vi "TCP-Com.vi"(8 "Exit Control Label":string="Exit Button", 9 "pwd":string, 10 "LabView Port":u16=4000, 11 "VI Refnum":refnum<vi>) -> (0 "error out":errorcluster)   [LabVIEW 2019]
doc: "This template is for the Queued Message Handler design pattern.\n\nThe Event Handling Loop generates messages based on user interface actions.\n\nThe Message Handling Loop processes messages generated by the Event Handling Loop, or by other messages. The messages are string values, so new messages can be added easily to the Message Cases case structure in the Message Handling Loop. Each message cluster can also provide an optional value for Message Data, which is a variant that can be converted to whatever message-specific data is required."
uses:
  support/TPC-Enum.ctl
  support/Message Queue/Enqueue Message (Single).vi
  <vilib>/Utility/error.llb/Error Cluster From Error Code.vi
  <vilib>/ErrorRing/Error Ring.xnode
  support/Message Queue/Message Queue.lvlib
  support/User Event - Stop/User Event - Stop.lvlib
  <vilib>/Utility/Data Type/NI_Data Type.lvlib
panel:
  out "connection ID":refnum<k5>
  out "Client Connected":bool
  in  "Request":string
  in  "Try request":bool
  in  "Exit":bool
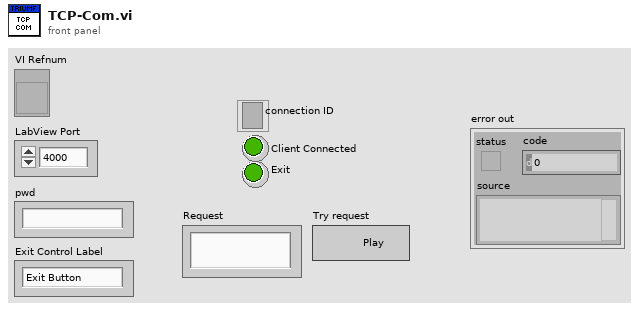
[diagram p1: front panel]
types:
  T1 = typedef "TPC-Enum.ctl" = enum16{"Wait For Client", "Check Client", "Listen"}
  T2 = typedef "Message Queue.lvlib/All Message Queues.ctl" = cluster{"TCP":refnum<queue>}
  T3 = typedef "NI_Data Type.lvlib/Data Type.ctl" = enum8{"Invalid Type", "Void", "I8", "I16", "I32", "I64", "U8", "U16", "U32", "U64", "Single Float", "Double Float", "Extended Float", "Single Complex", "Double Complex", "Extended Complex", "Enum U8", "Enum U16", "Enum U32", "Enum U64", "Single Float With Unit", "Double Float With Unit", "Extended Float With Unit", "Single Complex with Unit", "Double Complex with Unit", "Extended Complex with Unit", "Boolean", "String", "Path", "Picture", "Tag", "Array", "Cluster", "Variant", "LV Variant", "Waveform", "Timestamp", "Digital Waveform", "Digital Data", "ExpressData", "Refnum", "External Data", "VI", "Poly VI", "LabVIEW Class Instance", "Fixed Point", "Set Collection", "Map Collection"}
  T4 = enum16{"Standard", "Buffered", "CRLF", "Immediate"}
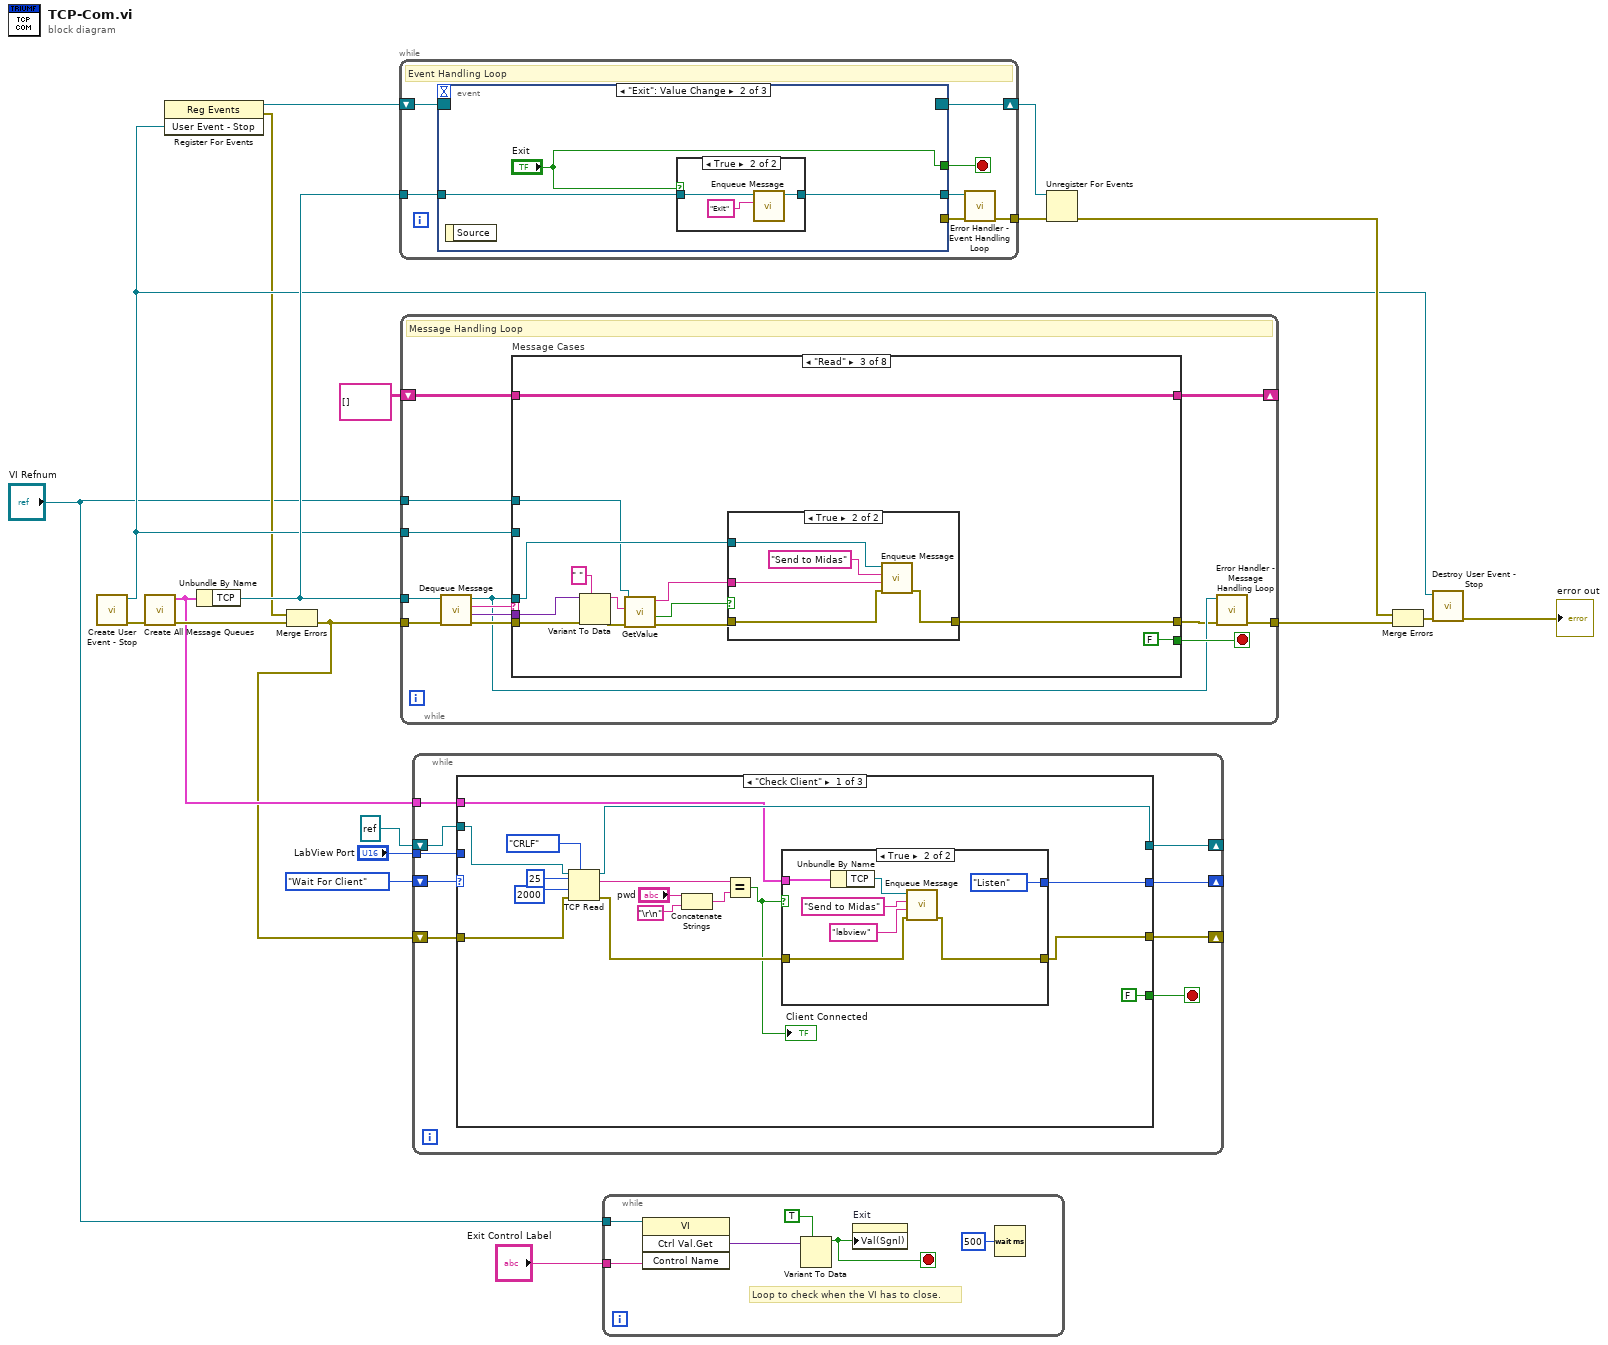
[diagram p0: block diagram]
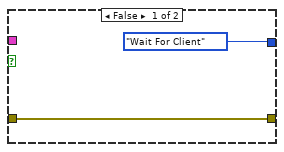
[diagram p2: hidden frame]
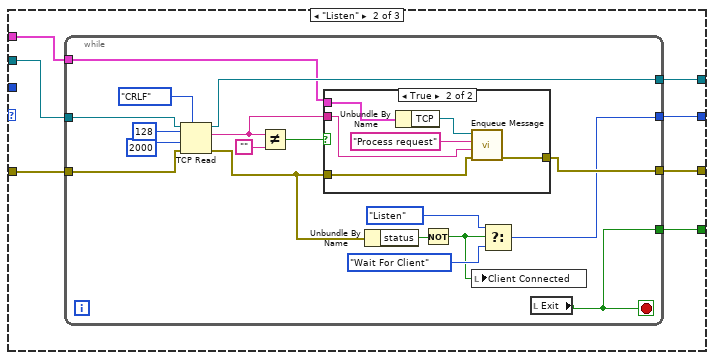
[diagram p3: hidden frame]
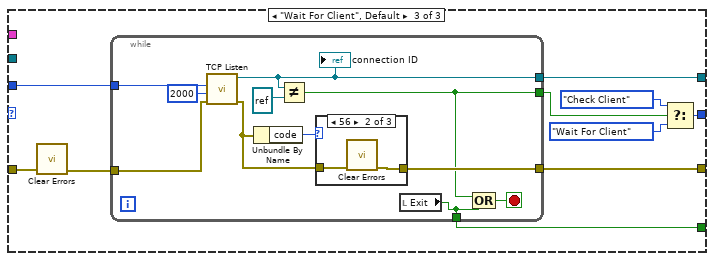
[diagram p5: hidden frame]
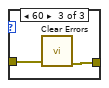
[diagram p7: hidden frame]
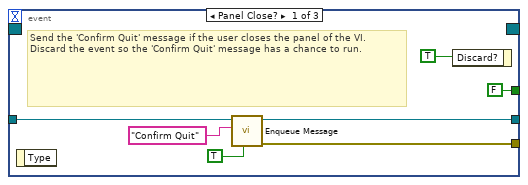
[diagram p8: hidden frame]
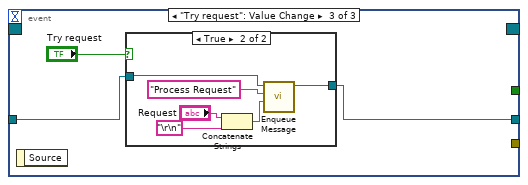
[diagram p10: hidden frame]
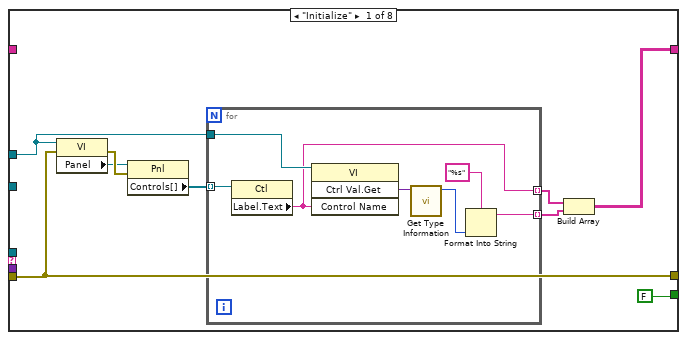
[diagram p12: hidden frame]
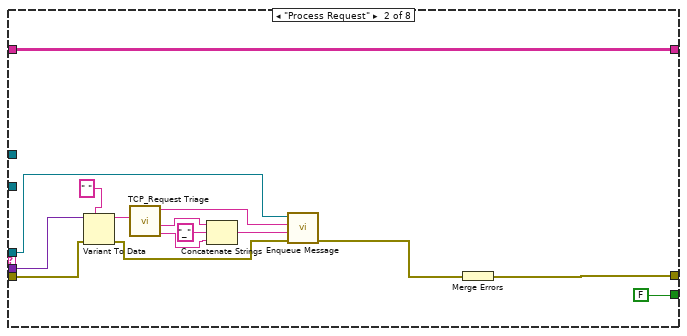
[diagram p13: hidden frame]
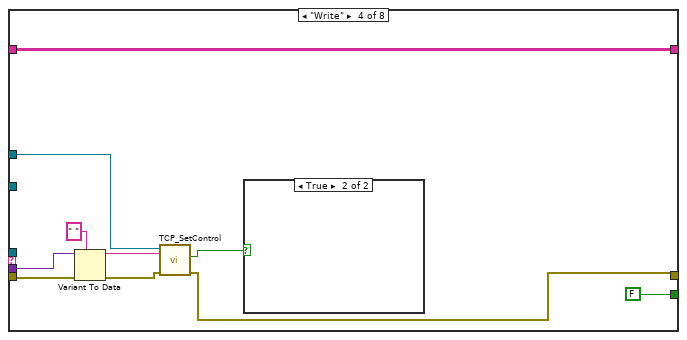
[diagram p15: hidden frame]
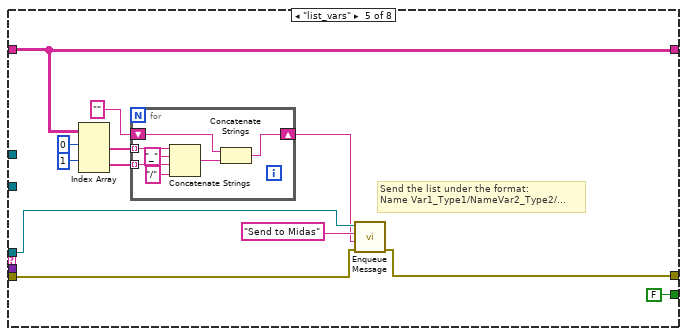
[diagram p17: hidden frame]
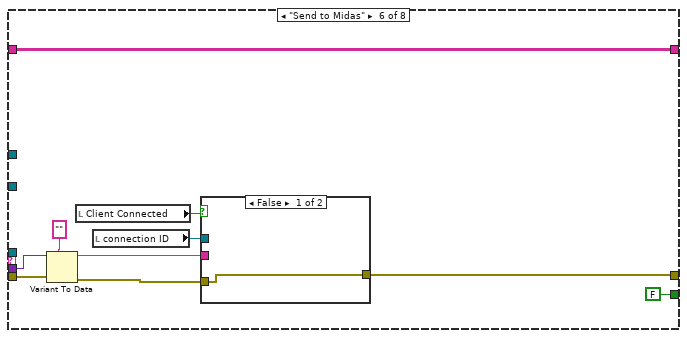
[diagram p18: hidden frame]
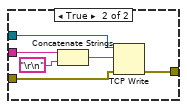
[diagram p19: hidden frame]
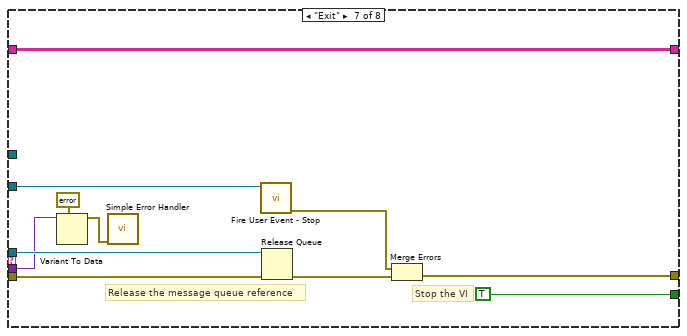
[diagram p20: hidden frame]
diagram:
  n1 = call "Create User Event - Stop.vi"() -> ("error out"=w17:errorcluster, "User Event - Stop"=w11:refnum<user-event>)  [unwired: 10 in]
  n2 = call "Create All Message Queues.vi"("error in (no error)"=w17) -> ("error out"=w20:errorcluster, "Message Queues out"=w6:T2)  [unwired: 9 in]
  n3 = register-events(w11) -> (reference out=w12:refnum<event-registration>, error out=w10:errorcluster)  [unwired: 2 in]
  n4 = Unbundle By Name(w6) -> ("TCP"=w18:refnum<queue>)
  n5 = Merge Errors(w10, w20) -> (w2:errorcluster)
  n6 = while {
    tunnel: w18 -> [w27]
    shift-right: [w25] -> w14
    shift-left: w12 -> [w26]
    tunnel: [w21] -> w13
    stop <- w23 stop-if-true
    # "Event Handling Loop"
    n7 = event shown="[1] \"Exit\": Value Change" {
      selector: w26 -> [_ _ _]
      dyn-events: [_ _ _] -> w25
      timeout: _ -> [_ _ _]
      tunnel: [FALSE ("Discard?") "Exit" _] -> w23
      tunnel: w27 -> [w33 w37 w43]
      tunnel: [w32 _ _] -> w24
      tunnel: [w31 w36 w42] -> w22
      event Panel Close? {
        # "Send the 'Confirm Quit' message if the user closes the panel of the VI. Discard the event so the 'Confirm Quit' message has a chance to run."
        n8 = event-data() -> ()  [unwired: 1 in, 1 out]
        n9 = call-poly "Enqueue Message.vi"("Priority Message? (F)"=TRUE, "Message"="Confirm Quit", "Message Queue"=w33) -> ("error out"=w32:errorcluster, "dup Message Queue"=w31:refnum<queue>)  [unwired: 7 in]
        n10 = event-data("Discard?"=TRUE) -> ()  [unwired: 1 in, 1 out]
      }
      event "Exit": Value Change {
        n11 = event-data() -> ()  [unwired: 1 in, 1 out]
        n12 = case shown="True" "Exit" {
          tunnel: w37 -> [w38 w41]
          tunnel: [w38 w39] -> w36
          frame False {
          }
          frame True {
            n13 = call-poly "Enqueue Message.vi"("Message"="Exit", "Message Queue"=w41) -> ("dup Message Queue"=w39:refnum<queue>)  [unwired: 8 in, 1 out]
          }
        }
      }
      event "Try request": Value Change {
        n14 = event-data() -> ()  [unwired: 1 in, 1 out]
        n15 = case shown="True" "Try request" {
          tunnel: w43 -> [w45 w50]
          tunnel: [w45 w49] -> w42
          frame False {
          }
          frame True {
            n16 = Concatenate Strings("Request", "\r\n") -> (w47:string)
            n17 = call-poly "Enqueue Message.vi"("Message Data"=w47, "Message"="Process Request", "Message Queue"=w50) -> ("dup Message Queue"=w49:refnum<queue>)  [unwired: 7 in, 1 out]
          }
        }
      }
    }
    n18 = call "Error Handler - Event Handling Loop.vi"("error in (no error)"=w24, "Message Queue"=w22) -> ("dup error in"=w21:errorcluster)  [unwired: 8 in, 1 out]
  }
  n19 = while {
    tunnel: w18 -> [w58]
    tunnel: w11 -> [w63]
    tunnel: w2 -> [w62]
    tunnel: [w56] -> w19
    tunnel: "VI Refnum" -> [w54]
    shift-right: [w53] -> _
    shift-left: string[][] [] -> [w52]
    stop <- w64 stop-if-true
    # "Message Handling Loop"
    n20 = call "Dequeue Message.vi"("error in (no error)"=w62, "Message Queue"=w58) -> ("error out"=w61:errorcluster, "Message Data"=w59:variant, "Message"=w60:string, "dup Message Queue"=w57:refnum<queue>)  [unwired: 6 in]
    n21 = case "Message Cases" shown="\"Read\"" w60 {
      selector: w60 -> [_ _ _ _ _ _ _ w174]
      tunnel: w57 -> [_ w88 w105 _ w135 _ w171 _]
      tunnel: w61 -> [w69 w93 w107 w123 w134 w151 w165 _]
      tunnel: [w69 w95 w104 w115 w133 w144 w168 w175] -> w55
      tunnel: [FALSE FALSE FALSE FALSE FALSE FALSE TRUE FALSE] -> w64
      tunnel: w59 -> [_ w94 w108 w122 _ w150 w162 _]
      tunnel: w63 -> [_ _ _ _ _ _ w167 _]
      tunnel: w54 -> [w68 _ w96 w118 _ _ _ _]
      tunnel: [w65 w81 w102 w120 w131 w153 w161 w172] -> w53
      tunnel: w52 -> [_ w81 w102 w120 w131 w153 w161 w172]
      frame "Initialize" {
        # "Initialize - All initialization work should take place in this message, since other loops can potentially enqueue messages that execute immediately after this one."
        n22 = property class="VI"(reference=w68, error in=w69) -> (error out=w72:errorcluster, "Panel"=w71:refnum<vi>)  [unwired: 1 out]
        n23 = property class="Pnl"(reference=w71, error in=w72) -> ("Controls[]"=w70:refnum<vi>[])  [unwired: 2 out]
        n24 = for {
          tunnel: w70 -> [w80] mode=indexing
          tunnel: w68 -> [w77]
          tunnel: [w75] -> w66 mode=indexing
          tunnel: [w74] -> w67 mode=indexing
          n25 = property class="Ctl"(reference=w80) -> ("Label.Text"=w74:string)  [unwired: 1 in, 2 out]
          n26 = invoke class="VI" method="Ctrl Val.Get"(reference=w77, "Control Name"=w74) -> ("Get Control Value Variant"=w76:variant)  [unwired: 2 in, 3 out]
          n27 = call <vilib>:"Get Type Information.vi"("variant"=w76) -> ("type"=w78:T3)  [unwired: 6 in, 4 out]
          n28 = Format Into String(format string="%s", w78) -> (resulting string=w75:string)  [unwired: 2 in, 1 out]
        }
        n29 = Build Array(w67, w66) -> (w65:string[][])
      }
      frame "Process Request" {
        # "Something - Replace this message with functionality for your own application."
        n30 = Variant To Data(error in=w93, type=" " ("Message"), Variant=w94) -> (data=w86:string, error out=w89:errorcluster)
        n31 = call "TCP_Request Triage.vi"("Message"=w86) -> ("Value"=w83:string, "Variable"=w84:string, "Request"=w85:string)  [unwired: 8 in]
        n32 = Concatenate Strings(w84, "_" ("string"), w83) -> (w87:string)
        n33 = call-poly "Enqueue Message.vi"("error in (no error)"=w89, "Message Data"=w87, "Message"=w85, "Message Queue"=w88) -> ("error out"=w90:errorcluster)  [unwired: 6 in, 1 out]
        n34 = Merge Errors(w90) -> (w95:errorcluster)
      }
      frame "Read" {
        n35 = Variant To Data(error in=w107, type=" " ("Message"), Variant=w108) -> (data=w97:string, error out=w101:errorcluster)
        n36 = call "GetValue.vi"("reference"=w96, "Input"=w97, "error in (no error)"=w101) -> ("Answer"=w99:string, "Found?"=w98:bool, "error out"=w100:errorcluster)  [unwired: 5 in]
        n37 = case shown="True" w98 {
          tunnel: [w109 w114] -> w104
          tunnel: w100 -> [w109 w113]
          tunnel: w105 -> [_ w112]
          tunnel: w99 -> [_ w110]
          frame False {
          }
          frame True {
            n38 = call-poly "Enqueue Message.vi"("error in (no error)"=w113, "Message Data"=w110, "Message"="Send to Midas", "Message Queue"=w112) -> ("error out"=w114:errorcluster)  [unwired: 6 in, 1 out]
          }
        }
      }
      frame "Write" {
        n39 = Variant To Data(error in=w123, type=" " ("Message"), Variant=w122) -> (data=w119:string, error out=w117:errorcluster)
        n40 = call "TCP_SetControl.vi"("VI Refnum"=w118, "Input"=w119, "error in (no error)"=w117) -> ("Found?"=w116:bool, "error out"=w115:errorcluster)  [unwired: 6 in]
        n41 = case shown="True" w116 {
          frame False {
          }
          frame True {
          }
        }
      }
      frame "list_vars" {
        # "Send the list under the format:\nName Var1_Type1/NameVar2_Type2/..."
        n42 = Index Array(array=w131, index (row) #1=0 ("index (row)"), index (row) #2=1 ("index (row)")) -> (element #1=w129:string[], element #2=w127:string[])  [unwired: 2 in]
        n43 = for {
          tunnel: w129 -> [w143] mode=indexing
          tunnel: w127 -> [w141] mode=indexing
          shift-right: [w137] -> w125
          shift-left: "" -> [w139]
          n44 = Concatenate Strings(w143, "_" ("string"), w141, "/" ("string")) -> (w138:string)
          n45 = Concatenate Strings(w139, w138) -> (w137:string)
        }
        n46 = call-poly "Enqueue Message.vi"("error in (no error)"=w134, "Message Data"=w125, "Message"="Send to Midas", "Message Queue"=w135) -> ("error out"=w133:errorcluster)  [unwired: 6 in, 1 out]
      }
      frame "Send to Midas" {
        n47 = Variant To Data(error in=w151, type="", Variant=w150) -> (data=w146:string, error out=w145:errorcluster)
        n48 = local read "Client Connected"() -> (w148:bool)
        n49 = local read "connection ID"() -> (w147:refnum<k5>)
        n50 = case shown="False" w148 {
          tunnel: w147 -> [_ w156]
          tunnel: w146 -> [_ w160]
          tunnel: w145 -> [w154 w157]
          tunnel: [w154 w155] -> w144
          frame False {
          }
          frame True {
            n51 = Concatenate Strings(w160, "\r\n") -> (w158:string)
            n52 = TCP Write(connection ID=w156, data in=w158, error in (no error)=w157) -> (error out=w155:errorcluster)  [unwired: 1 in, 2 out]
          }
        }
      }
      frame "Exit" {
        # "Stop the VI"
        # "Release the message queue reference"
        # "Exit - Exit the application."
        n53 = Variant To Data(type=errorcluster {"status"=FALSE, "code"=0, "source"=""} ("error constant"), Variant=w162) -> (data=w163:errorcluster)  [unwired: 1 in, 1 out]
        n54 = call <vilib>:"Simple Error Handler.vi"("error in (no error)"=w163) -> ()  [unwired: 4 in, 5 out]
        n55 = call "Fire User Event - Stop.vi"("User Event - Stop"=w167) -> ("error out"=w166:errorcluster)  [unwired: 10 in]
        n56 = Release Queue(queue=w171, error in (no error)=w165) -> (error out=w169:errorcluster)  [unwired: 1 in, 2 out]
        n57 = Merge Errors(w166, w169) -> (w168:errorcluster)
      }
      frame Default {
        # "'Default' case only runs if there is a message that isn't defined in any of the other cases.  Output a programming error."
        n58 = xnode "Error Ring"("parameter 0"=w174) -> ("error out"=w175:errorcluster)
      }
    }
    n59 = call "Error Handler - Message Handling Loop.vi"("error in (no error)"=w55, "Message Queue"=w57) -> ("dup error in"=w56:errorcluster)  [unwired: 8 in, 1 out]
  }
  n60 = while {
    shift-right: [w188] -> _
    shift-left: TPC-Enum."Wait For Client" -> [w191]
    tunnel: "LabView Port" -> [w190]
    shift-right: [w189] -> _
    shift-left: refnum<k5> refnum ("connection ID") -> [w184]
    shift-right: [w187] -> _
    shift-left: w2 -> [w186]
    tunnel: w6 -> [w183]
    stop <- w185 stop-if-true
    n61 = case shown="\"Check Client\"" w191 {
      tunnel: w190 -> [_ _ w258]
      tunnel: w186 -> [w204 w222 w250]
      tunnel: [w198 w221 w257] -> w189
      tunnel: [w195 w218 w253] -> w188
      tunnel: [FALSE w217 w252] -> w185
      tunnel: [w194 w219 w251] -> w187
      tunnel: w184 -> [w203 w223 _]
      tunnel: w183 -> [w197 w220 _]
      frame "Check Client" {
        n62 = TCP Read(connection ID=w203, bytes to read=25, error in (no error)=w204, 7:T4."CRLF" ("mode (standard)"), 9:2000 ("timeout ms (25000)")) -> (connection ID out=w198:refnum<k5>, data out=w200:string, error out=w196:errorcluster)
        n63 = Concatenate Strings("pwd", "\r\n") -> (w199:string)
        n64 = Equal?(x=w200, y=w199) -> (x = y?=w192:bool)
        "Client Connected" <- w192
        n65 = case shown="True" w192 {
          tunnel: w197 -> [_ w216]
          tunnel: w196 -> [w209 w212]
          tunnel: [TPC-Enum."Wait For Client" TPC-Enum."Listen"] -> w195
          tunnel: [w209 w210] -> w194
          frame False {
          }
          frame True {
            n66 = Unbundle By Name(w216) -> ("TCP"=w215:refnum<queue>)
            n67 = call-poly "Enqueue Message.vi"("error in (no error)"=w212, "Message Data"="labview", "Message"="Send to Midas", "Message Queue"=w215) -> ("error out"=w210:errorcluster)  [unwired: 6 in, 1 out]
          }
        }
      }
      frame "Listen" {
        n68 = while {
          tunnel: w223 -> [w238]
          tunnel: w222 -> [w237]
          tunnel: [w234] -> w221
          tunnel: w220 -> [w232]
          tunnel: [w231] -> w219
          tunnel: [w226] -> w218
          tunnel: [w225] -> w217
          stop <- w225 stop-if-true
          n69 = TCP Read(connection ID=w238, bytes to read=128, error in (no error)=w237, 7:T4."CRLF" ("mode (standard)"), 9:2000 ("timeout ms (25000)")) -> (connection ID out=w234:refnum<k5>, data out=w233:string, error out=w229:errorcluster)
          n70 = Not Equal?(x=w233, y="") -> (x != y?=w235:bool)
          n71 = case shown="True" w235 {
            tunnel: w233 -> [_ w245]
            tunnel: w232 -> [_ w246]
            tunnel: w229 -> [w242 w244]
            tunnel: [w242 w243] -> w231
            frame False {
            }
            frame True {
              n72 = Unbundle By Name(w246) -> ("TCP"=w248:refnum<queue>)
              n73 = call-poly "Enqueue Message.vi"("error in (no error)"=w244, "Message Data"=w245, "Message"="Process request", "Message Queue"=w248) -> ("error out"=w243:errorcluster)  [unwired: 6 in, 1 out]
            }
          }
          n74 = Unbundle By Name(w229) -> ("status"=w230:bool)
          n75 = Not(x=w230) -> (.not. x?=w224:bool)
          n76 = local write "Client Connected"(w224) -> ()
          n77 = Select(t=TPC-Enum."Listen", s=w224, f=TPC-Enum."Wait For Client") -> (s? t:f=w226:T1)
          n78 = local read "Exit"() -> (w225:bool)
        }
      }
      frame "Wait For Client", Default {
        n79 = call <vilib>:"Clear Errors.vi"("error in (no error)"=w250) -> ("error out"=w249:errorcluster)  [unwired: 5 in, 1 out]
        n80 = while {
          tunnel: w258 -> [w269]
          tunnel: w249 -> [w267]
          tunnel: [w260] -> w256
          tunnel: [w265] -> w257
          tunnel: [w262] -> w251
          tunnel: [w259] -> w252
          stop <- w261 stop-if-true
          n81 = call <vilib>:"TCP Listen.vi"("error in (no error)"=w267, "timeout ms (wait forever: -1)"=2000, "port"=w269) -> ("error out"=w263:errorcluster, "connection ID"=w265:refnum<k5>)  [unwired: 4 in, 3 out]
          "connection ID" <- w265
          n82 = Unbundle By Name(w263) -> ("code"=w264:i32)
          n83 = Not Equal?(x=w265, y=refnum<k5> refnum ("connection ID")) -> (x != y?=w260:bool)
          n84 = case shown="56" w264 {
            tunnel: w263 -> [w270 w272 w274]
            tunnel: [w270 w271 w273] -> w262
            frame 0, Default {
            }
            frame 56 {
              n85 = call <vilib>:"Clear Errors.vi"("error in (no error)"=w272) -> ("error out"=w271:errorcluster)  [unwired: 5 in, 1 out]
            }
            frame 60 {
              n86 = call <vilib>:"Clear Errors.vi"("error in (no error)"=w274) -> ("error out"=w273:errorcluster)  [unwired: 5 in, 1 out]
            }
          }
          n87 = local read "Exit"() -> (w259:bool)
          n88 = Compound Arithmetic op=OR(w260, w259) -> (w261:bool)
        }
        n89 = Select(t=TPC-Enum."Check Client", s=w256, f=TPC-Enum."Wait For Client") -> (s? t:f=w253:T1)
      }
    }
  }
  n90 = while {
    tunnel: "VI Refnum" -> [w275]
    tunnel: "Exit Control Label" -> [w276]
    stop <- w278 stop-if-true
    # "Loop to check when the VI has to close."
    n91 = invoke class="VI" method="Ctrl Val.Get"(reference=w275, "Control Name"=w276) -> ("Get Control Value Variant"=w277:variant)  [unwired: 2 in, 3 out]
    n92 = Variant To Data(type=TRUE, Variant=w277) -> (data=w278:bool)  [unwired: 1 in, 1 out]
    n93 = property on="Exit" class="Bool (strict)"("Val(Sgnl)"=w278) -> ()  [unwired: 2 in, 2 out]
    n94 = Wait (ms)(milliseconds to wait=u32 500) -> ()  [unwired: 1 out]
  }
  n95 = Unregister For Events(event registration refnum=w14, error in=w13) -> (error out=w15:errorcluster)
  n96 = Merge Errors(w15, w19) -> (w16:errorcluster)
  n97 = call "Destroy User Event - Stop.vi"("error in (no error)"=w16, "User Event - Stop"=w11) -> ("error out"=→"error out":errorcluster)  [unwired: 9 in]
